vi "FestoCPX.Station.ProdSuctionGripper.Set.vi"(6 "wait for product (F)":bool, 8 "error in":errorcluster, 9 "Sucker (0: Final)":i32, 10 "Position":T2, 11 "Slot":T1) -> (0 "error out":errorcluster, 2 "Product Present":bool)   [LabVIEW 2016]
uses:
  Station/Station.ValvePosition.ctl
  Station/Station.ProductSlot.ctl
  tools/Translator/Translator.Message.ctl
  Station/Station.ProductSuctionGripper.Type.ctl
  FestoCPX.DO.Signal.ctl
  FestoCPX.DI.Signal.ctl
  tools/EventLog/EventLog.EventSource.ctl
  FestoCPX.Valve(1out0in).vi
  FestoCPX.Valve(1out1in).vi
  tools/EventLog/EventLog.CreateError(array).vi
  tools/Wait (with error).vi
  tools/Translator/Translator.Translate.Status (NoError).vi
  tools/Translator/Translator.FormatMessage.vi
  FestoCPX.DO.Data.Set.vi
  FestoCPX.DI.Data.State.Get.vi
  FestoCPX.DI.Data.States.Get.vi
  tools/Translator/Translator.Global.vi
  tools/ErrorHandling/ErrorHandling.Create.vi
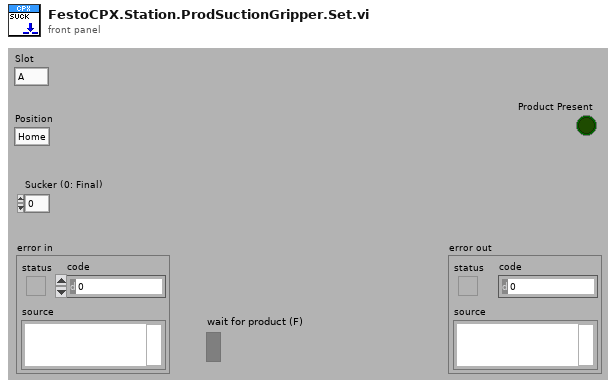
[diagram p1: front panel]
types:
  T1 = typedef "Station.ProductSlot.ctl" = enum8{"A", "B"}
  T2 = typedef "Station.ValvePosition.ctl" = enum16{"Home", "Work"}
  T3 = typedef "Station.ProductSuctionGripper.Type.ctl" = enum8{"Final A", "Final B", "Slot 1 A", "Slot 1 B", "Slot 2 A", "Slot 2 B", "Slot 3 A", "Slot 3 B", "Slot 4 A", "Slot 4 B"}
  T4 = typedef "Translator.Message.ctl" = enum16{"-", "Event confirmed", "Log out", "Log in", "Shutdown", "Cancel", "Start", "Begin time", "End time", "Duration", "Service Mode", "Ignore Results", "Serial Format", "On", "Off", "OK", "NOK", "NOK %s", "Home", "Work", "Close", "Open", "In progress...", "Missing", "Empty", "Hardware failure", "Initial", "Default", "Total", "Out of range", "Free disk space is below 1GB - contact technician", "Error %d >> %s", "Error %d >> %s >> %s", "Msg %d >> %s", "Laser msg %d %s", "Laser cmd error %s %d", "Laser cmd failed %s", "Laser cmd warning %s", "Laser disconnected", "Laser status %s", "Laser already started", "Laser job unkonwn %s", "Laser job missing %s", "Laser job select failure %s", "Unable to start laser printing (%s)", "Unable to stop laser printing (%s)", "Laser marking aborted", "Laser marking timeout", "Unable to reset Laser Interlock (%s)", "Unable to trigger Laser. Laser not ready (%s)", "Laser job '%s' coordinates not configured", "Starting %s", "Quitting %s", "Configured", "Initializing", "Quitting", "Loading", "Loaded %d results", "Loaded %d events", "Running", "Stopped", "Summary", "Laser", "Do you want to continue?", "Do you want to delete the configuration?", "The configuration is being used by an order. Unable to delete!", "Press confirm button", "Station is not based. Do you want to exit?", "Station requires changeover. Do you want to run the test?", "Test options are not set as default. Do you want to continue?", "Formatting of WabcoNo is disabled. Do you want to continue?", "Product not detected. Do you want to continue?", "Product scan failed. Do you want to continue?", "Calibration", "Log out?", "System", "All", "IDLE", "Translating...%s", "Not found", "Alarm %s", "Run", "Skip", "Abort", "Repeat", "Please wait...", "Database disconnected", "Database disconnected - changeover disabled!", "Login to database successful", "Login to database failed: %d; %s", "Unable to check the product status of reference %d - database disconnected", "Unable to set the product status of reference %d - database disconnected", "Variant file backup %s", "Read variant (%s)", "Result", "Station armed!", "Station requires changeover!", "Select reference number...", "EMERGENCY BUTTON - press Control button", "EMERGENCY DOOR - press Control button", "Resetting Emergency...", "Unable to reset safety circuit - Emergency Button pressed", "Unable to reset safety circuit - Emergency Side Door open", "Station not based", "Station based", "Station not empty", "Station basing...", "No order", "Press Start to begin new order", "Scanning new order", "Order NOK. Correct or scan again", "Order OK. Press Accept", "Order ready", "Revolver incorrect", "Fork incorrect", "Revolver missing", "Revolver empty", "Container missing", "Offline results", "Offline statistics", "Updating statistics %.1f %%", "DMC Configurator", "Door open", "Close the front door", "Press start button", "Done. Open the front door", "Running...", "Running...%.1f %%", "Pause %s", "Pause %s. NOK container missing", "Pause %s. OK container missing", "Pause %s. Revolver empty", "Pause %s. Revolver missing", "Pause %s. Revolver incorrect", "Pause %s. Fork missing", "Pause %s. Fork incorrect", "Pause %s. Too many failures", "Pause %s. Unloading failure", "Pause %s. One slot is not working", "Pause %s. Part order is done. Empty OK container", "Pause %s. Unable to move product to slot", "Pause %s. Unable to move back product pusher", "Pause %s. Unable to lift product", "Pause %s. Unable to move back product lifter", "Pause %s. Unable to move product arm to Work", "Pause %s. Unable to move product arm to NOK", "Pause %s. Unable to move product arm to OK", "Pause %s. Unable to unsuck the NOK product", "Pause %s. Unable to drop the NOK product", "Pause %s. Product OK missing", "Pause %s. Unable to unsuck the OK product", "Pause %s. Unable to drop the OK product", "Stopping...", "File '%s' is missing", "File '%s' is broken", "File '%s' is running", "Log file started (%s)", "Log file ended (%s)", "Log file stopped (%s)", "Log file ignored (%s)", "Log file exported (%s)", "Log file export failed (%s)", "Wrong serial number in log file", "Wrong reference number in log file", "Test steps are missing", "%s = %.3f", "Process param '%s' not found in DB", "Process param '%s' wrong order", "Process param '%s' value %.3f out of limits (%.3f; %.3f)", "Step%d param '%s' not found in DB", "Step%d param '%s' wrong order", "Step%d param '%s' value %.3f out of limits (%.3f; %.3f)", "Step%d EV '%s' not found in DB", "Step%d EV '%s' wrong order", "\"%s\" not found in DB", "\"%s\" wrong order", "\"%s\" value %.3f out of limits (%.3f; %.3f)", "\"%s\" not found in software", "Process init (%s)", "Process started", "Process restarted", "Process run", "Process done", "Process done - remove OK container", "Process aborted", "Process aborted at work", "Process aborted at home", "Process error", "Process error at home", "Process error at work", "Process close", "Process pause", "Process continue", "Process door open", "Process door close", "Process pause at slot %s due to %s", "Select plate from the order to process", "Do you want to start the process?", "Do you want to continue the process?", "There is unfinished order. Do you want to put the new order?", "Product %s %d OK", "Product %s %d NOK", "Unable to unload the slot %s. Product missing in the slot", "Unable to unload the slot %s. Product already in the arm", "Unable to accept the product as OK. Product missing in slot %s", "Unable to accept the product as OK. Product could not drop into the container at slot %s", "Unable to accept the product as NOK. Product could not drop into the container at slot %s", "Scan failed. Error %s", "Scan failed. Scanner disconnected", "Scan failed. Wrong Wabco number %d, limit (%d,%d)", "Scan failed. Wrong serial number %d, limit (%d,%d)", "Scan failed. Wrong date %d, limit (%d,%d)", "Scan failed. Wrong product wabco number %d (expected %d)", "Scan failed. Wrong product serial number %d (expected > 0)", "Scan OK %s", "Scan failed. Unable to determine table position (%s)", "Scan failed. Timeout", "Tune failed. Scanner disconnected", "Tune failed. Timeout", "%s = %d", "%s = %d->%d", "Unable to set %s = %.2f - Air Pressure Inside off", "Unable to set digital output '%s' = %d", "Unable to activate air pressure inside - timeout", "Unable to activate air pressure inside - aborted", "Unable to switch on Air Main Valve - Air Pressure Inlet off", "Unable to switch on Air Main Valve - Door open", "Unable to switch off Air Main Valve - timeout", "Unable to switch off Air Main Valve - aborted", "Unable to rotate Table - timeout", "Unable to rotate Table - aborted", "Unable to rotate Table - Product Move not in Home position", "Unable to rotate Table - Air Pressure Inside off", "Unable to rotate Table - Product Lift A not in Home position", "Unable to rotate Table - Product Lift B not in Home position", "Unable to rotate Table - unlock before movement timeout", "Unable to rotate Table - lock after movement timeout", "Unable to move Table Lock to %s position - timeout", "Unable to move Table Lock to %s position - aborted", "Unable to move Table Lock to %s position - Air Pressure Inside off", "Unable to move Table Lock to %s position - Table not in position", "Unable to move Product Lift A to %s position - timeout", "Unable to move Product Lift B to %s position - timeout", "Unable to move Product Lift A to %s position - aborted", "Unable to move Product Lift B to %s position - aborted", "Unable to move Product Lift A to %s position - Air Pressure Inside off", "Unable to move Product Lift B to %s position - Air Pressure Inside off", "Unable to move Product Lift A to %s position - Table not locked", "Unable to move Product Lift B to %s position - Table not locked", "Unable to move Product Lift A to %s position - Product Arm not in Work position", "Unable to move Product Lift B to %s position - Product Arm not in Work position", "Unable to set Product Suction Gripper %s to %s - timeout", "Unable to set Product Suction Gripper %s to %s - aborted", "Unable to set Product Suction Gripper %s to %s - Air Pressure Inside off", "Unable to set Product Suction Gripper %s to %s - Table slot unkown", "Unable to move Product Arm to %s position - timeout", "Unable to move Product Arm to %s position - aborted", "Unable to move Product Arm to %s position - Air Pressure Inside off", "Unable to move Product Arm to %s position - Product Lift A not in Home position", "Unable to move Product Arm to %s position - Product Lift B not in Home position", "Unable to move Product to %s position - timeout", "Unable to move Product to %s position - aborted", "Unable to move Product to %s position - Air Pressure Inside off", "Unable to move Product to %s position - Table not in position"}
  T5 = typedef "EventLog.EventSource.ctl" = enum16{"All", "Gui", "Ref", "File", "Arch", "Seq", "CPX", "DB", "Laser", "Scan.P", "Scan.O"}
  T6 = typedef "FestoCPX.DO.Signal.ctl" = enum16{"Safety Reset", "Air Main Valve", "Door Lock", "Button LED Start", "Button LED Stop", "Button LED Control", "Traffic LED Red", "Traffic LED Orange", "Traffic LED Green", "Horn", "Laser Interlock", "Laser Trigger", "Laser Fume Extractor", "Product Suction Gripper Slot 1 A", "Product Suction Gripper Slot 1 B", "Product Suction Gripper Slot 2 A", "Product Suction Gripper Slot 2 B", "Product Suction Gripper Slot 3 A", "Product Suction Gripper Slot 3 B", "Product Suction Gripper Slot 4 A", "Product Suction Gripper Slot 4 B", "Product Suction Gripper Final A", "Product Suction Gripper Final B", "Lamp", "Q1 Product Move Work", "Q1 Product Move Home", "Q2 Table Turn Work", "Q2 Table Turn Home", "Q3 Product Lift A", "Q3 Product Lift B", "Q4 Product Arm OK", "Q4 Product Arm NOK", "Q5 Product Arm Work", "Q6 Product BlowOut A", "Q6 Product BlowOut B"}
  T7 = typedef "FestoCPX.DI.Signal.ctl" = enum16{"S.C. Emergency Stop", "S.C. Side Door Close", "S.C. Front Door Close", "S.C. Front Door Secured", "Button Start", "Button Stop", "Button Control", "Product Move Home", "Product Move Work", "Table Position", "Table Lock", "Product Lift A Home", "Product Lift B Home", "Product Arm OK", "Product Arm NOK", "Product Arm Work", "Revolver ID 1", "Revolver ID 2", "Revolver ID 3", "Revolver ID 4", "Revolver ID 5", "Air Pressure Inside", "Air Pressure Inlet", "Product Slot 1 A Present", "Product Slot 1 B Present", "Product Slot 2 A Present", "Product Slot 2 B Present", "Product Slot 3 A Present", "Product Slot 3 B Present", "Product Slot 4 A Present", "Product Slot 4 B Present", "Product Final A Present", "Product Final B Present", "Product Output A Present", "Product Output B Present", "Product Container OK Present", "Product Container NOK Present", "Fork ID 1", "Fork ID 2"}
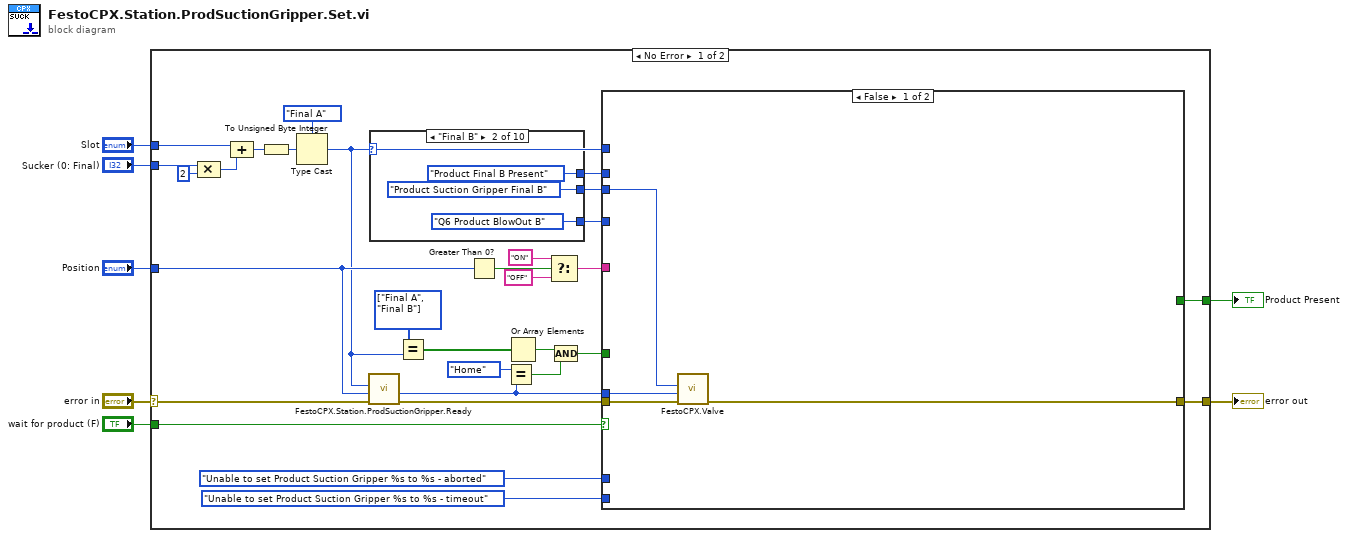
[diagram p0: block diagram]
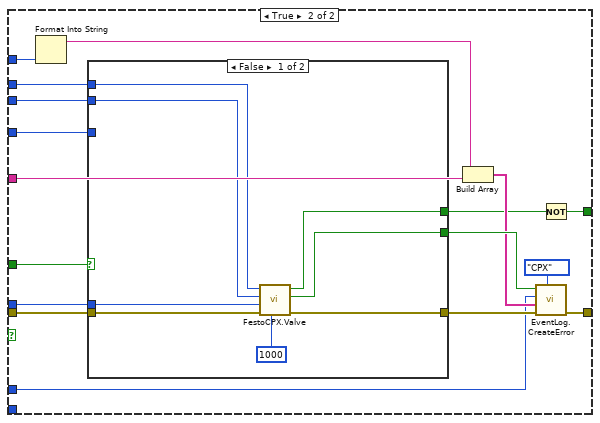
[diagram p2: hidden frame]
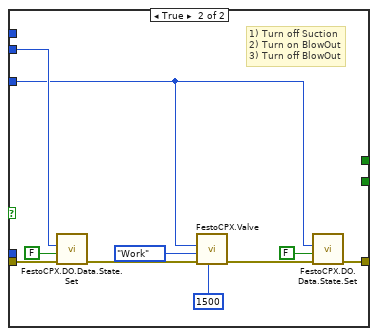
[diagram p3: hidden frame]
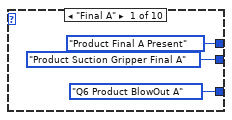
[diagram p4: hidden frame]
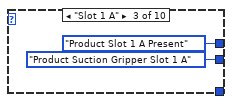
[diagram p5: hidden frame]
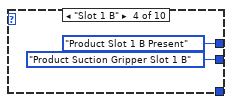
[diagram p6: hidden frame]
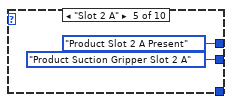
[diagram p7: hidden frame]
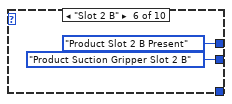
[diagram p8: hidden frame]
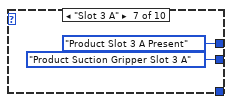
[diagram p9: hidden frame]
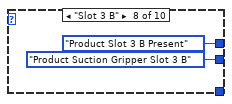
[diagram p10: hidden frame]
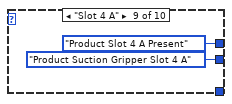
[diagram p11: hidden frame]
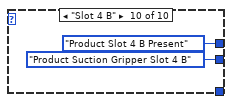
[diagram p12: hidden frame]
diagram:
  n1 = case shown="No Error" "error in" {
    selector: "error in" -> [w18 w98]
    tunnel: [w36 w98] -> w7
    tunnel: "Position" -> [w15 _]
    tunnel: "Sucker (0: Final)" -> [w19 _]
    tunnel: "Slot" -> [w35 _]
    tunnel: "wait for product (F)" -> [w34 _]
    tunnel: [w33 _] -> w1
    frame No Error {
      w14 = T3[] [enum."Final A", enum."Final B"] items=["Final A", "Final B", "Slot 1 A", "Slot 1 B", "Slot 2 A", "Slot 2 B", "Slot 3 A", "Slot 3 B", "Slot 4 A", "Slot 4 B"]
      n2 = Compound Arithmetic op=MULTIPLY(w19, 2 ("value")) -> (w20:i32)
      n3 = Compound Arithmetic op=ADD(w35, w20) -> (w23:i32)
      n4 = To Unsigned Byte Integer(number=w23) -> (unsigned 8bit integer=w22:u8)
      n5 = Type Cast(type=Station.ProductSuctionGripper.Type."Final A" ("Type"), x=w22) -> (*(type *) &x=w13:T3)
      n6 = call "FestoCPX.Station.ProdSuctionGripper.Ready.vi"("error in"=w18, "Position"=w15, "Type"=w13) -> ("error out"=w17:errorcluster)  [unwired: 7 in, 1 out]
      n7 = case shown="\"Final B\"" w13 {
        tunnel: [FestoCPX.DO.Signal."Product Suction Gripper Final A" ("CPX.DO") FestoCPX.DO.Signal."Product Suction Gripper Final B" ("CPX.DO") FestoCPX.DO.Signal."Product Suction Gripper Slot 1 A" ("CPX.DO") FestoCPX.DO.Signal."Product Suction Gripper Slot 1 B" ("CPX.DO") FestoCPX.DO.Signal."Product Suction Gripper Slot 2 A" ("CPX.DO") FestoCPX.DO.Signal."Product Suction Gripper Slot 2 B" ("CPX.DO") FestoCPX.DO.Signal."Product Suction Gripper Slot 3 A" ("CPX.DO") FestoCPX.DO.Signal."Product Suction Gripper Slot 3 B" ("CPX.DO") FestoCPX.DO.Signal."Product Suction Gripper Slot 4 A" ("CPX.DO") FestoCPX.DO.Signal."Product Suction Gripper Slot 4 B" ("CPX.DO")] -> w31
        tunnel: [FestoCPX.DI.Signal."Product Final A Present" ("DI") FestoCPX.DI.Signal."Product Final B Present" ("DI") FestoCPX.DI.Signal."Product Slot 1 A Present" ("DI") FestoCPX.DI.Signal."Product Slot 1 B Present" ("DI") FestoCPX.DI.Signal."Product Slot 2 A Present" ("DI") FestoCPX.DI.Signal."Product Slot 2 B Present" ("DI") FestoCPX.DI.Signal."Product Slot 3 A Present" ("DI") FestoCPX.DI.Signal."Product Slot 3 B Present" ("DI") FestoCPX.DI.Signal."Product Slot 4 A Present" ("DI") FestoCPX.DI.Signal."Product Slot 4 B Present" ("DI")] -> w30
        tunnel: [FestoCPX.DO.Signal."Q6 Product BlowOut A" ("CPX.DO") FestoCPX.DO.Signal."Q6 Product BlowOut B" ("CPX.DO") _ _ _ _ _ _ _ _] -> w8
        frame "Final A" {
        }
        frame "Final B" {
        }
        frame "Slot 1 A" {
        }
        frame "Slot 1 B" {
        }
        frame "Slot 2 A" {
        }
        frame "Slot 2 B" {
        }
        frame "Slot 3 A" {
        }
        frame "Slot 3 B" {
        }
        frame "Slot 4 A" {
        }
        frame "Slot 4 B" {
        }
      }
      n8 = Equal?(x=w14, y=w13) -> (x = y?=w12:bool[])
      n9 = Greater Than 0?(x=w15) -> (x > 0?=w25:bool)
      n10 = Equal?(x=Station.ValvePosition."Home", y=w15) -> (x = y?=w11:bool)
      n11 = Or Array Elements(Boolean array=w12) -> (logical OR=w10:bool)
      n12 = Select(t="ON" ("resulting string"), s=w25, f="OFF" ("resulting string")) -> (s? t:f=w27:string)
      n13 = Compound Arithmetic op=AND(w10, w11) -> (w9:bool)
      n14 = case shown="False" w34 {
        tunnel: [w38 w44] -> w36
        tunnel: Translator.Message."Unable to set Product Suction Gripper %s to %s - timeout" ("msg") -> [_ _]
        tunnel: w31 -> [w37 w57]
        tunnel: w30 -> [_ w56]
        tunnel: w17 -> [w40 w55]
        tunnel: w27 -> [_ w53]
        tunnel: Translator.Message."Unable to set Product Suction Gripper %s to %s - aborted" ("msg") -> [_ w48]
        tunnel: w15 -> [w39 w43]
        tunnel: w13 -> [_ w47]
        tunnel: [_ w45] -> w33
        tunnel: w9 -> [_ w42]
        tunnel: w8 -> [_ w41]
        frame False {
          n15 = call-poly "FestoCPX.Valve.vi"("error in (no error)"=w40, "Position"=w39, "Output"=w37) -> ("error out"=w38:errorcluster)  [unwired: 8 in]
        }
        frame True {
          n16 = Format Into String(w47) -> (resulting string=w54:string)  [unwired: 3 in, 1 out]
          n17 = case shown="False" w42 {
            tunnel: w57 -> [w65 w72]
            tunnel: w56 -> [w64 _]
            tunnel: w55 -> [w63 w74]
            tunnel: [w62 _] -> w51
            tunnel: [w61 w69] -> w50
            tunnel: [w60 _] -> w46
            tunnel: w43 -> [w58 _]
            tunnel: w41 -> [_ w67]
            frame False {
              n18 = call-poly "FestoCPX.Valve.vi"("Timeout [ms] (5000)"=u32 1000, "error in (no error)"=w63, "Position"=w58, "Output"=w65, "Input"=w64) -> ("error out"=w61:errorcluster, "Aborted?"=w62:bool, "Timeout?"=w60:bool)  [unwired: 4 in]
            }
            frame True {
              # "1) Turn off Suction\n2) Turn on BlowOut\n3) Turn off BlowOut"
              n19 = call "FestoCPX.DO.Data.State.Set.vi"("error in (no error)"=w74, "State"=FALSE, "CPX.DO"=w72) -> ("error out"=w73:errorcluster)  [unwired: 8 in]
              n20 = call-poly "FestoCPX.Valve.vi"("Timeout [ms] (0)"=u32 1500 ("Timeout [ms] (5000)"), "error in (no error)"=w73, "Position"=Station.ValvePosition."Work", "Output"=w67) -> ("error out"=w70:errorcluster)  [unwired: 7 in]
              n21 = call "FestoCPX.DO.Data.State.Set.vi"("error in (no error)"=w70, "State"=FALSE, "CPX.DO"=w67) -> ("error out"=w69:errorcluster)  [unwired: 8 in]
            }
          }
          n22 = Build Array(w54, w53) -> (w49:string[])
          n23 = call-poly "EventLog.CreateError.vi"("Source (All)"=EventLog.EventSource."CPX", "error in"=w50, "args"=w49, "msg"=w48, "create (T)"=w51) -> ("error out"=w44:errorcluster)  [unwired: 5 in, 1 out]
          n24 = Not(x=w46) -> (.not. x?=w45:bool)
        }
      }
    }
    frame Error {
    }
  }
  "error out" <- w7
  "Product Present" <- w1
